vi "startMission.vi"(8 "error in (no error)":errorcluster, 11 "GenericMission in":refnum<class "GenericMission.lvclass">) -> (0 "error out":errorcluster, 3 "GenericMission out":refnum<class "GenericMission.lvclass">)   [LabVIEW 2011, in "GenericMission.lvclass"]
doc: "Performs a start-up sequence for a mission. This method should always be called once a new mission has begun.\n\nNote: This is a dynamic dispatch method of GenericMission. The correct method will be called based on the run-time class of this object, a child class of GenericMission.\n\nAuthor: Jared Kirschner"
uses:
  GenericMission.lvclass
  2 Globals/2 Message Logger.vi
  Logger/Logger.lvclass
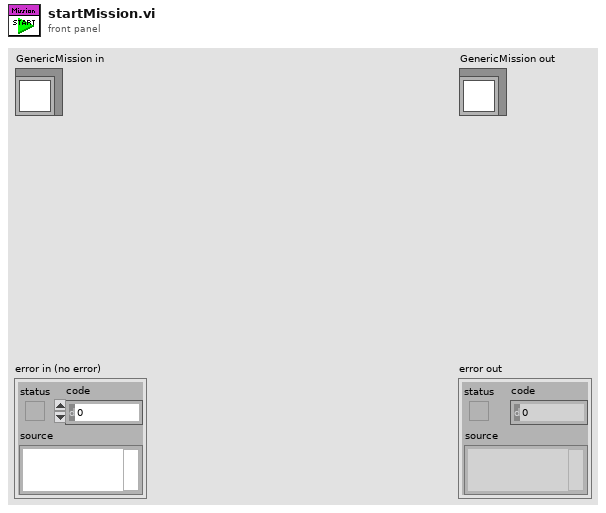
[diagram p1: front panel]
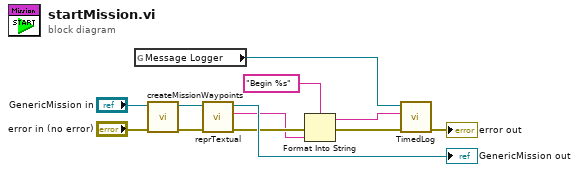
[diagram p0: block diagram]
diagram:
  n1 = global read "2 Message Logger.vi" "Message Logger"() -> (w10:refnum<class "Logger.lvclass">)
  n2 = call-dynamic "createMissionWaypoints.vi"("error in (no error)"="error in (no error)", "GenericMission in"="GenericMission in") -> ("error out"=w7:errorcluster, "GenericMission out"=w8:refnum<class "GenericMission.lvclass">)  [unwired: 8 in]
  n3 = call-dynamic "reprTextual.vi"("error in (no error)"=w7, "GenericMission in"=w8) -> ("error out"=w5:errorcluster, "Description"=w2:string, "GenericMission out"=→"GenericMission out":refnum<class "GenericMission.lvclass">)  [unwired: 7 in]
  n4 = Format Into String(format string="Begin %s", error in=w5, w2) -> (resulting string=w1:string, error out=w4:errorcluster)  [unwired: 1 in]
  n5 = call "TimedLog.vi"("error in (no error)"=w4, "Message"=w1, "Logger in"=w10) -> ("error out"=→"error out":errorcluster)  [unwired: 6 in, 2 out]
